vi "Set Data.vi"(9 "AOAIRefs":T1[](array[typedef]), 10 "Connector Type":T2, 11 "Data":T3) -> (1 "data changed":bool, 3 "Data out":T3)   [LabVIEW 2020, in "PXISlotGP.xctl"]
uses:
  PXISlotGP.xctl
  Data.ctl
  PXISlot XControl/Connector Type.ctl
  AOAIRefs.ctl
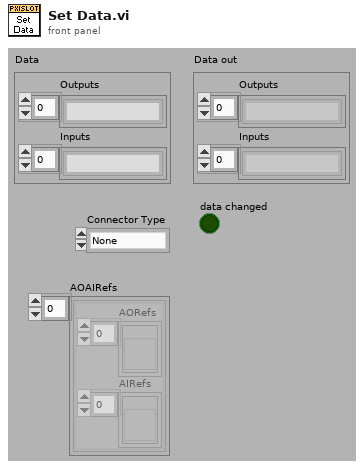
[diagram p1: front panel]
types:
  T1 = typedef "AOAIRefs.ctl" = cluster{"AORefs":refnum<vi>[], "AIRefs":refnum<vi>[]}
  T2 = typedef "Connector Type.ctl" = enum16{"None", "PXI-4461", "BNC-2110", "BNC-2090", "PXIe-4463", "PXIe-4464"}
  T3 = typedef "PXISlotGP.xctl/Data.ctl" = cluster{"Outputs":string[], "Inputs":string[]}
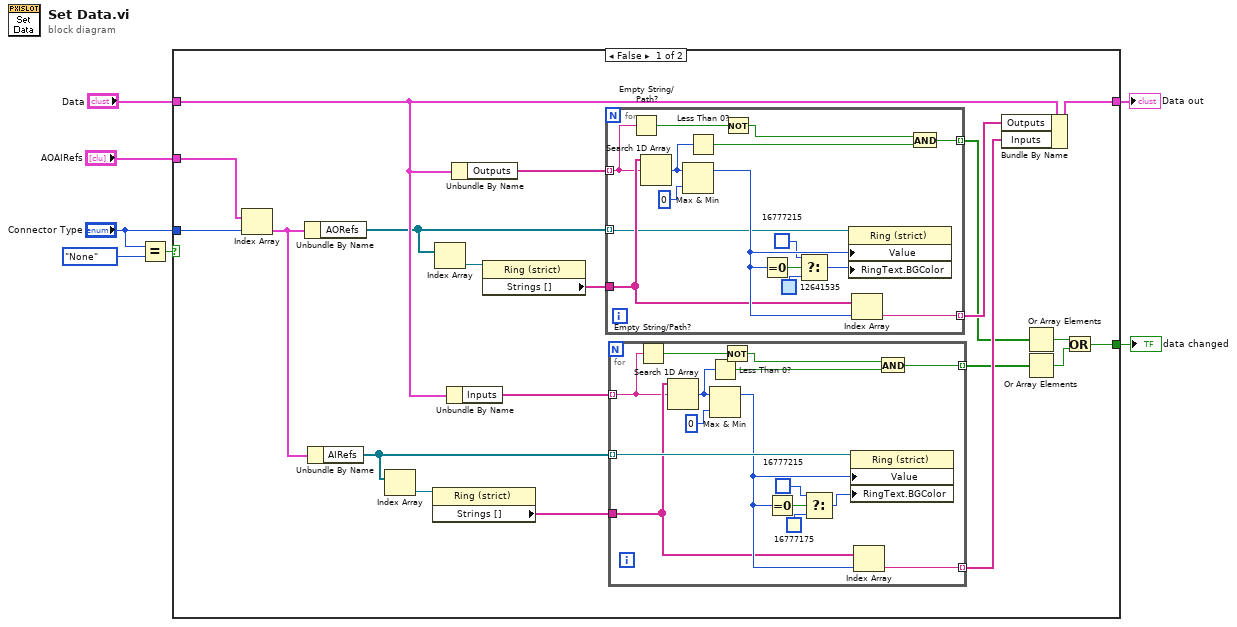
[diagram p0: block diagram]
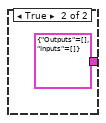
[diagram p2: hidden frame]
diagram:
  n1 = Equal?(x="Connector Type", y=Connector_Type."None") -> (x = y?=w5:bool)
  n2 = case shown="False" w5 {
    tunnel: "Data" -> [w26 _]
    tunnel: [w25 T3 {"Outputs"=[], "Inputs"=[]} ("Data")] -> w6
    tunnel: "Connector Type" -> [w24 _]
    tunnel: "AOAIRefs" -> [w20 _]
    tunnel: [w8 _] -> w1
    frame False {
      n3 = Index Array(array=w20, index=w24) -> (element=w19:T1)
      n4 = Unbundle By Name(w19) -> ("AORefs"=w16:refnum<vi>[])
      n5 = Unbundle By Name(w19) -> ("AIRefs"=w14:refnum<vi>[])
      n6 = Index Array(array=w14) -> (element=w15:refnum<vi>)  [unwired: 1 in]
      n7 = property class="Ring (strict)"(reference=w15) -> ("Strings []"=w13:string[])  [unwired: 1 in, 2 out]
      n8 = Index Array(array=w16) -> (element=w18:refnum<vi>)  [unwired: 1 in]
      n9 = Unbundle By Name(w26) -> ("Inputs"=w22:string[])
      n10 = Unbundle By Name(w26) -> ("Outputs"=w27:string[])
      n11 = property class="Ring (strict)"(reference=w18) -> ("Strings []"=w17:string[])  [unwired: 1 in, 2 out]
      n12 = for {
        tunnel: w27 -> [w31] mode=indexing
        tunnel: w16 -> [w35] mode=indexing
        tunnel: [w33] -> w23 mode=indexing
        tunnel: w17 -> [w36]
        tunnel: [w32] -> w12 mode=indexing
        n13 = Empty String/Path?(string/path=w31) -> (empty?=w29:bool)
        n14 = Search 1D Array(1D array=w36, element=w31) -> (index of element=w34:i32)  [unwired: 1 in]
        n15 = Max & Min(x=w34, y=0) -> (max(x,y)=w42:i32)  [unwired: 1 out]
        n16 = Less Than 0?(x=w34) -> (x < 0?=w30:bool)
        n17 = Not(x=w29) -> (.not. x?=w28:bool)
        n18 = Equal To 0?(x=w42) -> (x = 0?=w41:bool)
        n19 = Select(t=u32 16777215, s=w41, f=u32 12641535) -> (s? t:f=w39:u32)
        n20 = property class="Ring (strict)"(reference=w35, "Value"=w42, "RingText.BGColor"=w39) -> ()  [unwired: 1 in, 2 out]
        n21 = Index Array(array=w36, index=w42) -> (element=w33:string)
        n22 = And(x=w28, y=w30) -> (x .and. y?=w32:bool)
      }
      n23 = for {
        tunnel: w22 -> [w44] mode=indexing
        tunnel: w14 -> [w56] mode=indexing
        tunnel: [w48] -> w21 mode=indexing
        tunnel: w13 -> [w50]
        tunnel: [w46] -> w11 mode=indexing
        n24 = Empty String/Path?(string/path=w44) -> (empty?=w45:bool)
        n25 = Search 1D Array(1D array=w50, element=w44) -> (index of element=w49:i32)  [unwired: 1 in]
        n26 = Less Than 0?(x=w49) -> (x < 0?=w47:bool)
        n27 = Max & Min(x=w49, y=0) -> (max(x,y)=w52:i32)  [unwired: 1 out]
        n28 = Not(x=w45) -> (.not. x?=w43:bool)
        n29 = Equal To 0?(x=w52) -> (x = 0?=w55:bool)
        n30 = Select(t=u32 16777215, s=w55, f=u32 16777175) -> (s? t:f=w53:u32)
        n31 = property class="Ring (strict)"(reference=w56, "Value"=w52, "RingText.BGColor"=w53) -> ()  [unwired: 1 in, 2 out]
        n32 = Index Array(array=w50, index=w52) -> (element=w48:string)
        n33 = And(x=w43, y=w47) -> (x .and. y?=w46:bool)
      }
      n34 = Bundle By Name(cluster=w26, "Outputs"=w23, "Inputs"=w21) -> (w25:T3)
      n35 = Or Array Elements(Boolean array=w12) -> (logical OR=w10:bool)
      n36 = Or Array Elements(Boolean array=w11) -> (logical OR=w9:bool)
      n37 = Or(x=w10, y=w9) -> (x .or. y?=w8:bool)
    }
    frame True {
    }
  }
  "Data out" <- w6
  "data changed" <- w1
